vi "Destroy.vi"(8 "Error In":errorcluster, 11 "SFTP Attributes":refnum<class "SFTP Attributes.lvclass">) -> (0 "Error Out":errorcluster, 3 "lv-libssh2 Shared Library":path)   [LabVIEW 2018, in "Toolkit.lvlib" / "SFTP Attributes.lvclass"]
uses:
  SFTP Attributes.lvclass
  SFTP Attributes.lvclass/SFTP Attributes.ctl
  Toolkit.lvlib
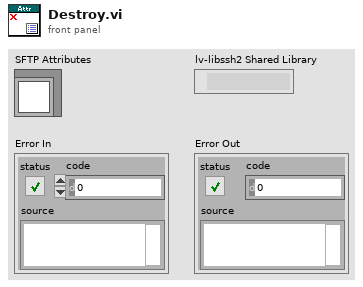
[diagram p1: front panel]
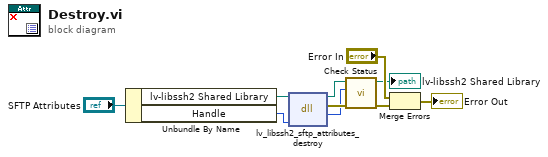
[diagram p0: block diagram]
diagram:
  n1 = Unbundle By Name("SFTP Attributes") -> ("lv-libssh2 Shared Library"=w8:path, "Handle"=w7:u64)
  n2 = dll-call lib="lv-libssh2.*" fn="lv_libssh2_sftp_attributes_destroy"(path in=w8, "handle"=w7) -> (path out=w5:path, error out=w6:errorcluster, "status"=w4:i32)  [unwired: 3 in]
  n3 = call "Check Status.vi"("Error In"=w6, "Status"=w4, "lv-libssh2 Shared Library In"=w5) -> ("Error Out"=w3:errorcluster, "lv-libssh2 Shared Library Out"=→"lv-libssh2 Shared Library":path)  [unwired: 7 in]
  n4 = Merge Errors("Error In", w3) -> (→"Error Out":errorcluster)
